vi "Write system_index.vi"(10 "system_index":i32, 11 "Heater in":refnum<class "Heater.lvclass">) -> (3 "Heater out":refnum<class "Heater.lvclass">)   [LabVIEW 2019, in "Heating.lvlib" / "Heater.lvclass"]
uses:
  Heater.lvclass
  Heater.lvclass/Heater.ctl
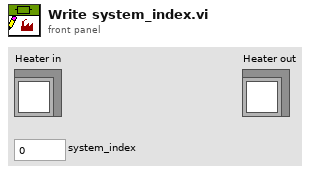
[diagram p1: front panel]
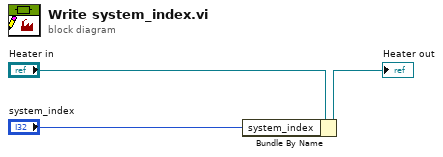
[diagram p0: block diagram]
diagram:
  n1 = Bundle By Name(cluster="Heater in", "system_index"="system_index") -> (→"Heater out":refnum<class "Heater.lvclass">)
